vi "HA4_yufan_dong.vi"(8 "Error In":errorcluster, 10 "LED Channel     (<device>/<port>/line0:7 )":tag="Dev1/port0/line0:1", 11 "Input Channel AI    (<device>/ai0:1 )":tag="Dev1/ai0") -> (0 "Error Out":errorcluster, 1 "Waveform Chart":cluster{"Waveform":dbl, "Waveform":dbl}[](graph), 2 "Digital":T1, 3 "Soll AO0":dbl format="%#.2g")   [LabVIEW 2021]
doc: "This is a traffic light system. It realized the output with hard device or simulated device. The light has four phases."
uses:
  Controls/digital_number_display_yufan_dong.ctl
  <vilib>/DAQmx/read.llb/DAQmx Read (Analog 2D DBL NChan NSamp).vi
  <vilib>/DAQmx/write.llb/DAQmx Write (Analog DBL 1Chan 1Samp).vi
  <vilib>/DAQmx/write.llb/DAQmx Write (Digital 1D Bool 1Chan 1Samp).vi
  <vilib>/DAQmx/create/channels.llb/DAQmx Create Channel (DO-Digital Output).vi
  <vilib>/DAQmx/create/channels.llb/DAQmx Create Channel (AI-Voltage-Basic).vi
  <vilib>/DAQmx/configure/timing.llb/DAQmx Timing (Sample Clock).vi
  <vilib>/DAQmx/create/channels.llb/DAQmx Create Channel (AO-Voltage-Basic).vi
  <vilib>/DAQmx/miscellaneous.llb/DAQmx Fill In Error Info.vi
panel:
  in  "Max Voltage":dbl=10.0
  in  "Min Voltage":dbl
  in  "Output Channel AO ( <device>/ao0 )":tag="Dev1/ao0"
  out "Delay (ms)":u32
  out "Sample Rate (Hz)":dbl=50.0
  in  "Stop":bool
  # "Note & Guide\n\n<<<<<< Channels >>>>>\n\nInput Channel\n<device>/ai0:1\neg. myDAQ1/ai0:1\n\nOutput Channel\n<device>/ao0\neg. myDAQ1/ao0\n\nLED Channel\n<device>/<port>/line0:7\neg. myDAQ1/port0/line0:7\n\n\nNotice: The AO0 interface must have the ability to recieve signal  0-10Volt, Because the Sollwert is 0-10V. \n\n\n\n\n\n<<<<<<< Others >>>>>>\n\nSample Rate 100Hz\nDelay 100ms\n\nDisplay might have Font-Problem\n\nAuthor\nYufan Dong - 15.Oct.2021"
  # "Using Input to Control and Display"
  # "Ist AI1"
  # "Ist AI0"
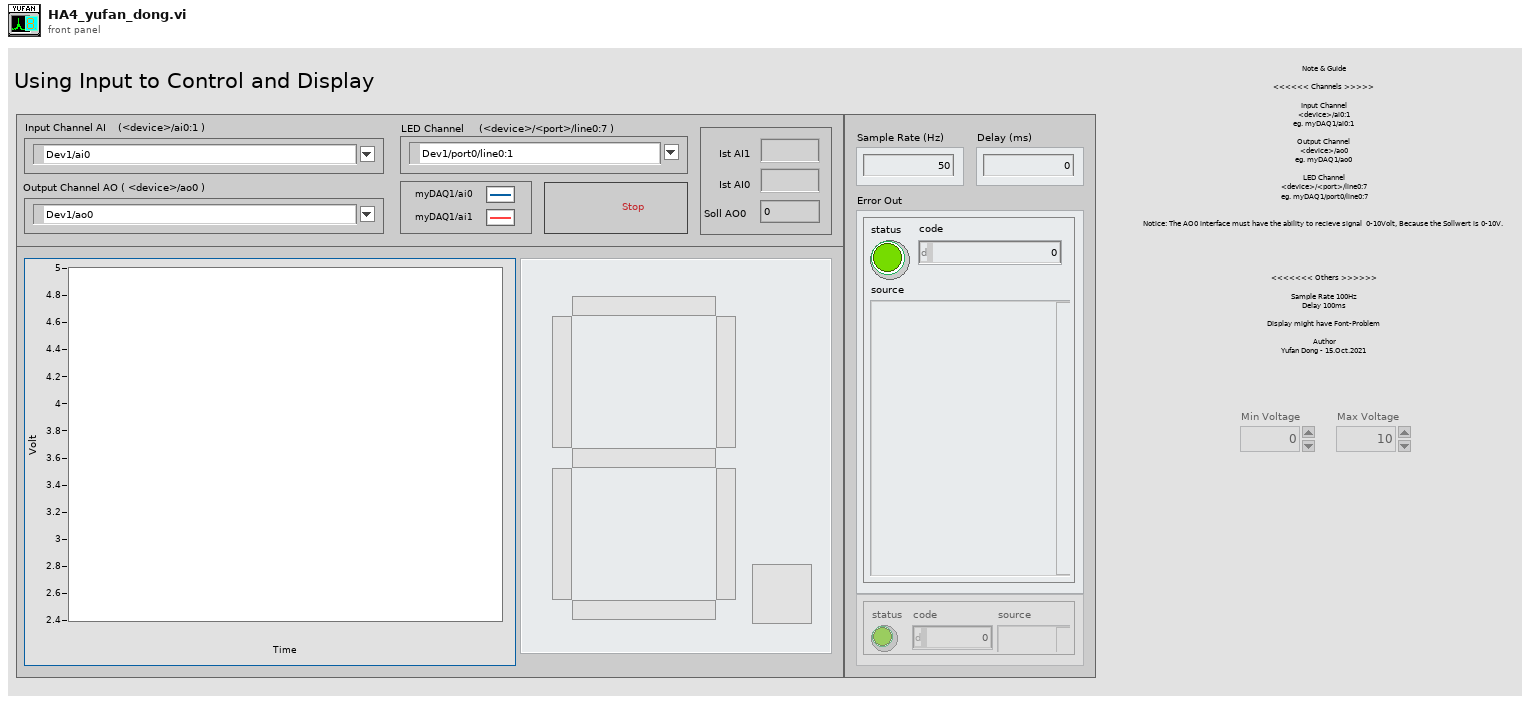
[diagram p1: front panel]
types:
  T1 = typedef "digital_number_display_yufan_dong.ctl" = cluster{"A":bool, "B":bool, "C":bool, "D":bool, "E":bool, "F":bool, "G":bool, "DP":bool}
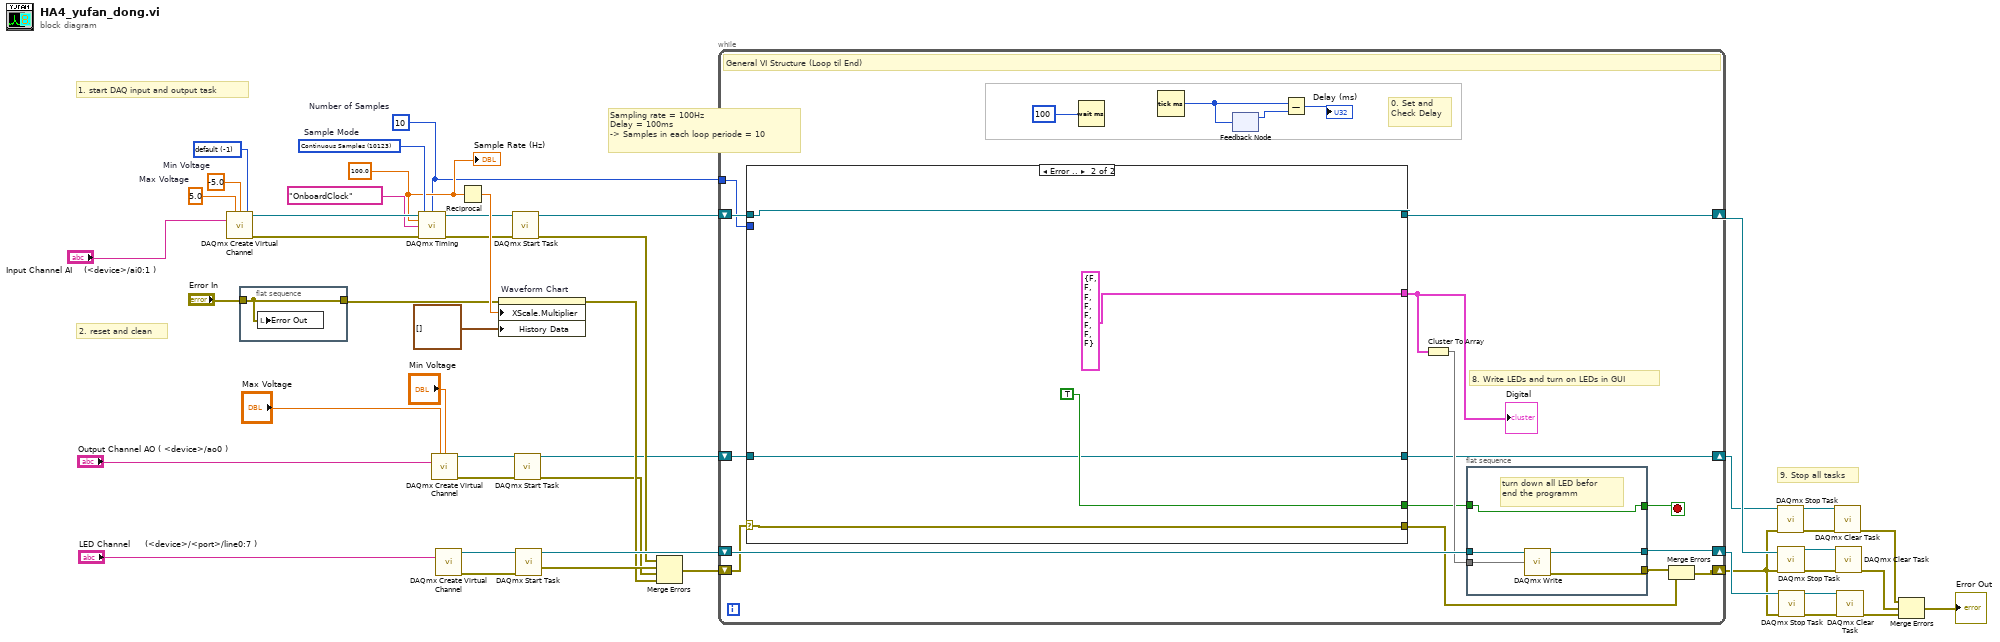
[diagram p0: block diagram]
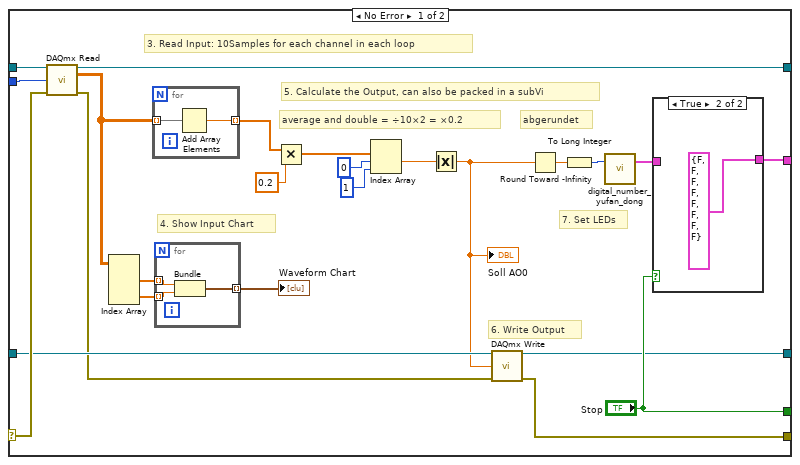
[diagram p2: hidden frame]
diagram:
  w29 = 100.0 ("Sample Rate")
  w34 = -1 items=["default"=-1, "RSE"=10083, "NRSE"=10078, "Differential"=10106, "Pseudodifferential"=12529] ("Terminal Configuration")
  w18 = 10  # Number of Samples
  w37 = 5.0  # Max Voltage
  w38 = -5.0  # Min Voltage
  w43 = 10123 items=["Finite Samples"=10178, "Continuous Samples"=10123, "Hardware Timed Single Point"=12522]  # Sample Mode
  # "Sampling rate = 100Hz\nDelay = 100ms\n-> Samples in each loop periode = 10"
  # "9. Stop all tasks"
  # "1. start DAQ input and output task"
  # "2. reset and clean"
  n1 = call-poly <vilib>:"DAQmx Create Virtual Channel.vi"("maximum value"=w37, "minimum value"=w38, "input terminal configuration"=w34, "physical channels"="Input Channel AI    (<device>/ai0:1 )") -> ("task out"=w41:refnum<k21>, "error out"=w42:errorcluster)  [unwired: 10 in]
  n2 = flat-sequence {
    tunnel: "Error In" -> [w47]
    tunnel: [w47] -> w1
    frame #0 {
      n3 = local write "Error Out"(w47) -> ()
    }
  }
  n4 = call-poly <vilib>:"DAQmx Timing.vi"("task/channels in"=w41, "sample mode"=w43, "samples per channel"=w18, "rate"=w29, "source"=tag "OnboardClock" ("Sample Clock Source"), "error in"=w42) -> ("task out"=w17:refnum<k21>, "error out"=w16:errorcluster)  [unwired: 8 in]
  n5 = call-poly <vilib>:"DAQmx Create Virtual Channel.vi"("maximum value"="Max Voltage", "minimum value"="Min Voltage", "physical channels"="Output Channel AO ( <device>/ao0 )") -> ("task out"=w14:refnum<k21>, "error out"=w15:errorcluster)  [unwired: 11 in]
  n6 = call-poly <vilib>:"DAQmx Create Virtual Channel.vi"("lines"="LED Channel     (<device>/<port>/line0:7 )") -> ("task out"=w44:refnum<k21>, "error out"=w45:errorcluster)  [unwired: 13 in]
  n7 = Reciprocal(x=w29) -> (1/x=w21:dbl)
  n8 = property on="Waveform Chart" class="WFChart (strict)"(error in=w1, "XScale.Multiplier"=w21, "History Data"=cluster{dbl, dbl}[] []) -> (error out=w10:errorcluster)  [unwired: 1 in, 1 out]
  n9 = call <vilib>:"DAQmx Start Task.vi"("task/channels in"=w17, "error in"=w16) -> ("task out"=w40:refnum<k21>, "error out"=w26:errorcluster)  [unwired: 12 in]
  n10 = call <vilib>:"DAQmx Start Task.vi"("task/channels in"=w14, "error in"=w15) -> ("task out"=w8:refnum<k21>, "error out"=w9:errorcluster)  [unwired: 12 in]
  n11 = call <vilib>:"DAQmx Start Task.vi"("task/channels in"=w44, "error in"=w45) -> ("task out"=w32:refnum<k21>, "error out"=w25:errorcluster)  [unwired: 12 in]
  n12 = Merge Errors(w26, w25, w9, w10) -> (w24:errorcluster)
  n13 = while {
    shift-right: [w60] -> w28
    shift-left: w40 -> [w61]
    shift-right: [w65] -> w27
    shift-left: w32 -> [w66]
    shift-right: [w51] -> w5
    shift-left: w24 -> [w55]
    tunnel: w18 -> [w59]
    shift-right: [w48] -> w4
    shift-left: w8 -> [w49]
    stop <- w53 stop-if-true
    # "8. Write LEDs and turn on LEDs in GUI"
    # "0. Set and \nCheck Delay"
    # "General VI Structure (Loop til End)"
    n14 = case shown="Error .." w55 {
      selector: w55 -> [w85 w106]
      tunnel: w61 -> [w95 w107]
      tunnel: [w94 w107] -> w60
      tunnel: [w73 w106] -> w50
      tunnel: w59 -> [w91 _]
      tunnel: [w82 T1 {"A"=FALSE, "B"=FALSE, "C"=FALSE, "D"=FALSE, "E"=FALSE, "F"=FALSE, "G"=FALSE, "DP"=FALSE} ("Digital")] -> w58
      tunnel: ["Stop" TRUE] -> w54
      tunnel: w49 -> [w76 w103]
      tunnel: [w75 w103] -> w48
      frame No Error {
        # "7. Set LEDs"
        # "6. Write Output"
        # "5. Calculate the Output, can also be packed in a subVi"
        # "4. Show Input Chart"
        # "abgerundet"
        # "average and double = ÷10×2 = ×0.2"
        # "3. Read Input: 10Samples for each channel in each loop"
        n15 = call-poly <vilib>:"DAQmx Read.vi"("task/channels in"=w95, "number of samples per channel"=w91, "error in"=w85) -> ("task out"=w94:refnum<k21>, "data"=w81:dbl[][], "error out"=w74:errorcluster)  [unwired: 10 in]
        n16 = Index Array(array=w81) -> (element #1=w80:dbl[], element #2=w79:dbl[])  [unwired: 4 in]
        n17 = for {
          tunnel: w81 -> [w102] mode=indexing
          tunnel: [w101] -> w89 mode=indexing
          n18 = Add Array Elements(numeric array=w102) -> (sum=w101:dbl)
        }
        n19 = for {
          tunnel: w80 -> [w98] mode=indexing
          tunnel: w79 -> [w97] mode=indexing
          tunnel: [w96] -> w78 mode=indexing
          n20 = Bundle("Waveform"=w98, "Waveform"=w97) -> (w96:cluster{"Waveform":dbl, "Waveform":dbl})  [unwired: 1 in]
        }
        "Waveform Chart" <- w78
        n21 = Multiply(x=w89, y=0.2) -> (x*y=w87:dbl[])
        n22 = Index Array(array=w87, index #1=0, index #2=1) -> (element #1=w77:dbl)  [unwired: 1 out]
        n23 = Absolute Value(x=w77) -> (abs(x)=w72:dbl)
        "Soll AO0" <- w72
        n24 = call-poly <vilib>:"DAQmx Write.vi"("task/channels in"=w76, "data"=w72, "error in"=w74) -> ("task out"=w75:refnum<k21>, "error out"=w73:errorcluster)  [unwired: 10 in, 1 out]
        n25 = Round Toward -Infinity(1:w72) -> (0:w90:dbl)
        n26 = To Long Integer(number=w90) -> (32bit integer=w88:i32)
        n27 = call "digital_number_yufan_dong.vi"("Numeric Control"=w88) -> ("Digital"=w83:T1)  [unwired: 2 in]
        n28 = case shown="True" "Stop" {
          tunnel: w83 -> [w99 _]
          tunnel: [w99 T1 {"A"=FALSE, "B"=FALSE, "C"=FALSE, "D"=FALSE, "E"=FALSE, "F"=FALSE, "G"=FALSE, "DP"=FALSE} ("Digital")] -> w82
          frame False {
          }
          frame True {
          }
        }
      }
      frame Error {
      }
    }
    "Digital" <- w58
    n29 = Wait (ms)(milliseconds to wait=u32 100) -> ()  [unwired: 1 out]
    n30 = Tick Count (ms)() -> (millisecond timer value=w63:u32)
    n31 = feedback #1() -> (w64:u32)  [unwired: 1 in]
    n32 = feedback-in #1(w63) -> ()
    n33 = Subtract(x=w63, y=w64) -> (x-y=→"Delay (ms)":u32)
    n34 = Cluster To Array(cluster=w58) -> (array=w57:bool[])
    n35 = flat-sequence {
      tunnel: w66 -> [w71]
      tunnel: [w70] -> w65
      tunnel: [w69] -> w52
      tunnel: w57 -> [w68]
      tunnel: w54 -> [w67]
      tunnel: [w67] -> w53
      frame #0 {
        # "turn down all LED befor \nend the programm"
        n36 = call-poly <vilib>:"DAQmx Write.vi"("task/channels in"=w71, "data"=w68) -> ("task out"=w70:refnum<k21>, "error out"=w69:errorcluster)  [unwired: 11 in, 1 out]
      }
    }
    n37 = Merge Errors(w52, w50) -> (w51:errorcluster)
  }
  n38 = call <vilib>:"DAQmx Stop Task.vi"("task/channels in"=w4, "error in"=w5) -> ("task out"=w7:refnum<k21>, "error out"=w6:errorcluster)  [unwired: 12 in]
  n39 = call <vilib>:"DAQmx Stop Task.vi"("task/channels in"=w28, "error in"=w5) -> ("task out"=w35:refnum<k21>, "error out"=w36:errorcluster)  [unwired: 12 in]
  n40 = call <vilib>:"DAQmx Stop Task.vi"("task/channels in"=w27, "error in"=w5) -> ("task out"=w31:refnum<k21>, "error out"=w30:errorcluster)  [unwired: 12 in]
  n41 = call <vilib>:"DAQmx Clear Task.vi"("task in"=w7, "error in"=w6) -> ("error out"=w3:errorcluster)  [unwired: 13 in]
  n42 = call <vilib>:"DAQmx Clear Task.vi"("task in"=w35, "error in"=w36) -> ("error out"=w23:errorcluster)  [unwired: 13 in]
  n43 = call <vilib>:"DAQmx Clear Task.vi"("task in"=w31, "error in"=w30) -> ("error out"=w22:errorcluster)  [unwired: 13 in]
  n44 = Merge Errors(w3, w23, w22) -> (→"Error Out":errorcluster)
  "Sample Rate (Hz)" <- w29
